vi "Send_Get_1Bit.vi"(8 "error in (no error)":errorcluster, 10 "Channel":u8, 11 "Serial Device in":refnum<class "Serial Device.lvclass">) -> (0 "error out":errorcluster, 2 "buffer":string, 3 "Serial Device out":refnum<class "Serial Device.lvclass">)   [LabVIEW 2019, in "Serial Device.lvclass"]
uses:
  Serial Device.lvclass
  Serial Device.lvclass/Serial Device.ctl
  0713ec9a-b44c-44ab-a500-c5f2b92f772c.vi
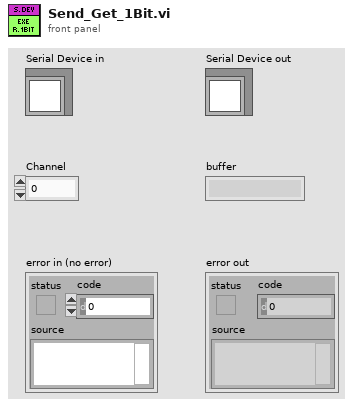
[diagram p1: front panel]
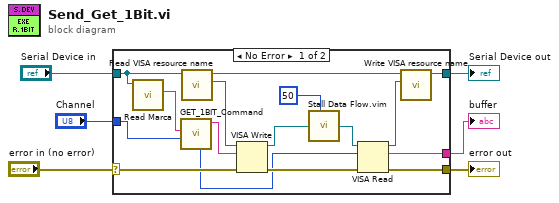
[diagram p0: block diagram]
diagram:
  n1 = case shown="No Error" "error in (no error)" {
    selector: "error in (no error)" -> [w20 w24]
    tunnel: [w16 w24] -> w5
    tunnel: [w12 w23] -> w3
    tunnel: "Serial Device in" -> [w22 w23]
    tunnel: "Channel" -> [w10 _]
    tunnel: [w11 _] -> w1
    frame No Error {
      n2 = call "Read Marca.vi"("Serial Device in"=w22) -> ("Marca"=w9:string)  [unwired: 8 in, 2 out]
      n3 = call "GET_1BIT_Command.vi"("Canal"=w10, "Marca"=w9) -> ("Command"=w7:string, "Bytes Expected"=w8:u32)  [unwired: 6 in, 2 out]
      n4 = call "Read VISA resource name.vi"("Serial Device in"=w22) -> ("VISA resource name"=w21:refnum<visa-resource-name>, "Serial Device out"=w13:refnum<class "Serial Device.lvclass">)  [unwired: 8 in, 1 out]
      n5 = VISA Write(VISA resource name=w21, write buffer=w7, error in (no error)=w20) -> (VISA resource name out=w19:refnum<visa-resource-name>, error out=w17:errorcluster)  [unwired: 1 out]
      n6 = call "Stall Data Flow.vim"("value in"=w19, "milliseconds to wait"=u32 50) -> ("value out"=w18:refnum<visa-resource-name>)  [unwired: 1 out]
      n7 = VISA Read(VISA resource name=w18, byte count=w8, error in (no error)=w17) -> (VISA resource name out=w14:refnum<visa-resource-name>, read buffer=w11:string, error out=w16:errorcluster)  [unwired: 1 out]
      n8 = call "Write VISA resource name.vi"("VISA resource name"=w14, "Serial Device in"=w13) -> ("Serial Device out"=w12:refnum<class "Serial Device.lvclass">)  [unwired: 8 in, 1 out]
    }
    frame Error {
    }
  }
  "error out" <- w5
  "Serial Device out" <- w3
  "buffer" <- w1
